vi "TEST_LoadConfigFile.vi"   [LabVIEW 2024]
uses:
  Control Definitions/Registry Keys.ctl
types:
  T1 = typedef "Registry Keys.ctl" = enum16{"Report Files Key", "Config Files Key"}
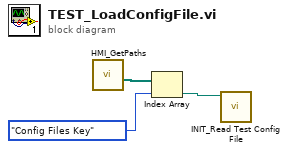
[diagram p0: block diagram]
diagram:
  n1 = call "HMI_GetPaths.vi"() -> ("Remote Paths"=w3:path[])  [unwired: 10 in, 1 out]
  n2 = Index Array(array=w3, index=Registry_Keys."Config Files Key" ("Reg Key")) -> (element=w1:path)
  n3 = call "INIT_Read Test Config File.vi"("Path"=w1) -> ()  [unwired: 9 in, 2 out]
